vi "Render Section.vi"(6 "Loader":refnum<class "Loader.lvclass">, 8 "Error In":errorcluster, 10 "Section":refnum<class "Section.lvclass">, 11 "Context In":refnum<class "Context.lvclass">) -> (0 "Error Out":errorcluster, 2 "Output":string, 3 "Context Out":refnum<class "Context.lvclass">)   [LabVIEW 2018, in "Toolkit.lvlib"]
uses:
  Toolkit.lvlib
  Context/Context.lvclass
  Nodes/Section/Section.lvclass
  Loaders/Loader/Loader.lvclass
  Nodes/Section/Section.lvclass/Section.ctl
  Data/Array/Array.lvclass
  Data/Array/Array.lvclass/Array.ctl
  Context/Context.lvclass/Context.ctl
  Data/Boolean/Boolean.lvclass
  Data/Function/Function.lvclass
  Data/String/String.lvclass
  Data/String/String.lvclass/String.ctl
  Data/Path/Path.lvclass
  Data/Path/Path.lvclass/Path.ctl
  Data/Datum/Datum.lvclass
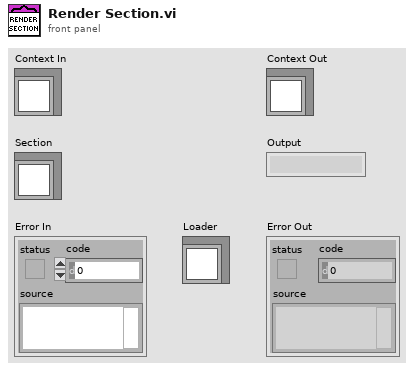
[diagram p1: front panel]
types:
  T1 = typedef "Toolkit.lvlib/Data.lvlib/Types.ctl" = enum16{"Array", "Boolean", "Function", "Map", "Null", "Pair", "Path", "String", "Unknown"}
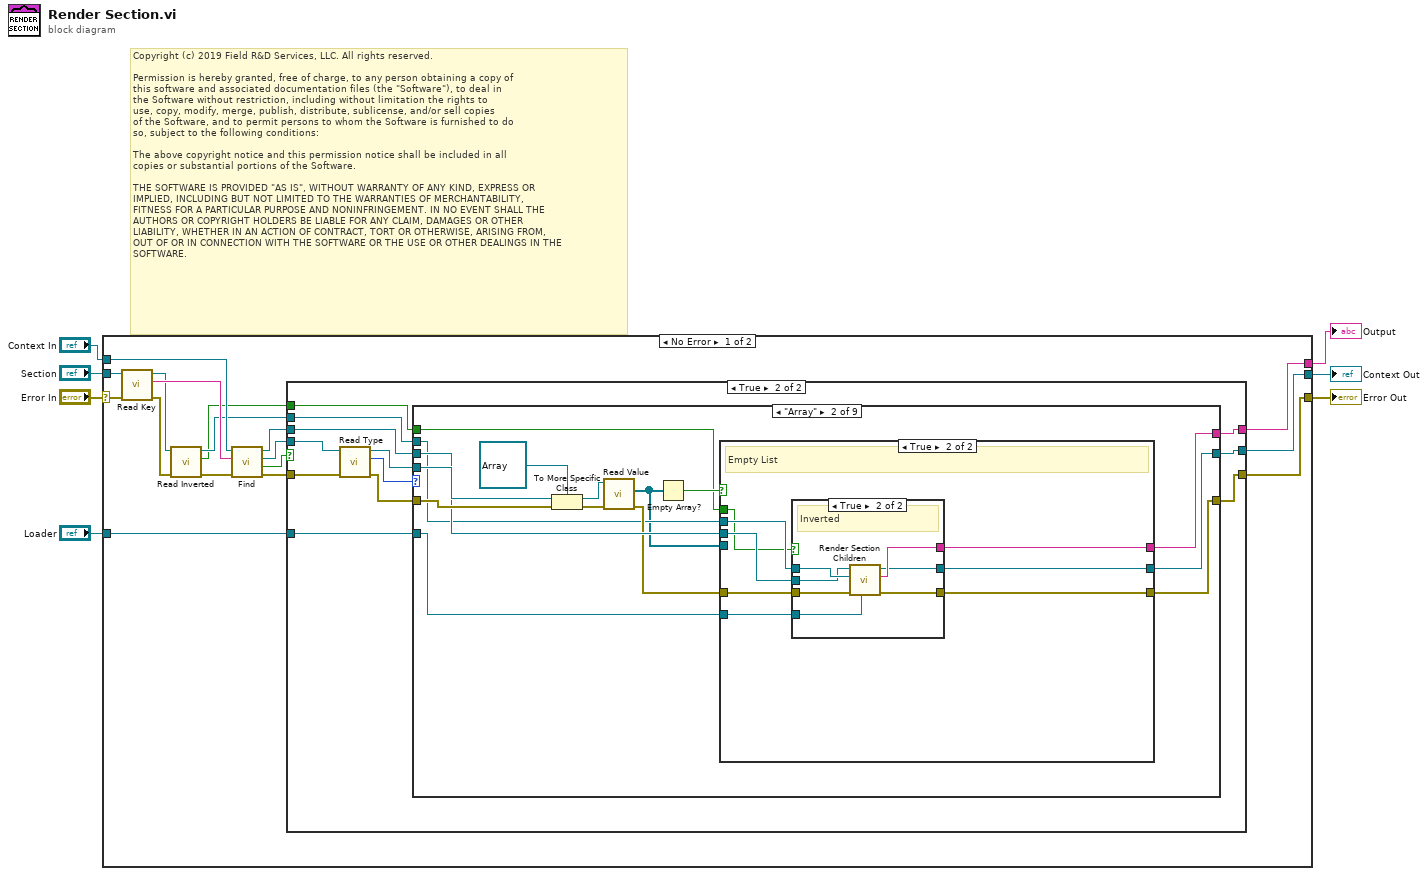
[diagram p0: block diagram]
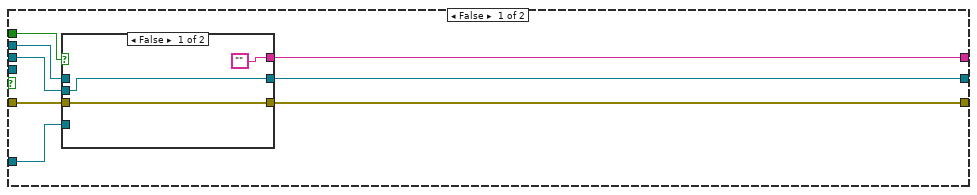
[diagram p2: hidden frame]
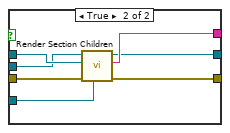
[diagram p3: hidden frame]
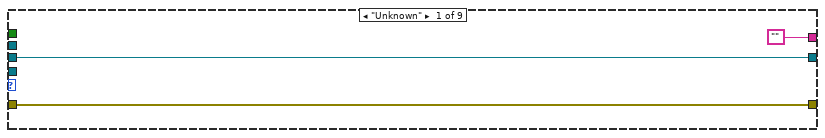
[diagram p4: hidden frame]
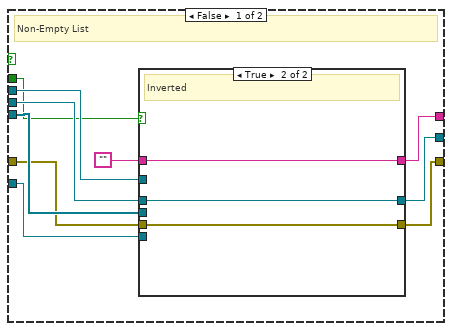
[diagram p5: hidden frame]
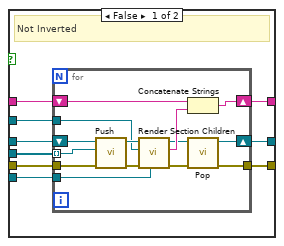
[diagram p6: hidden frame]
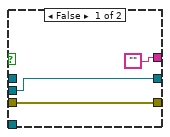
[diagram p7: hidden frame]
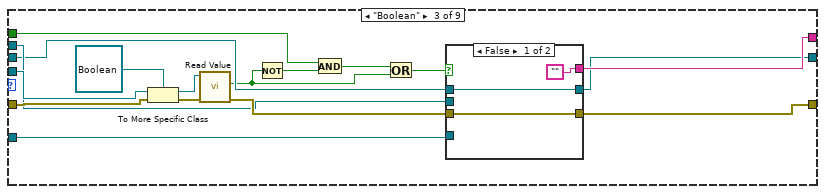
[diagram p8: hidden frame]
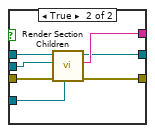
[diagram p9: hidden frame]
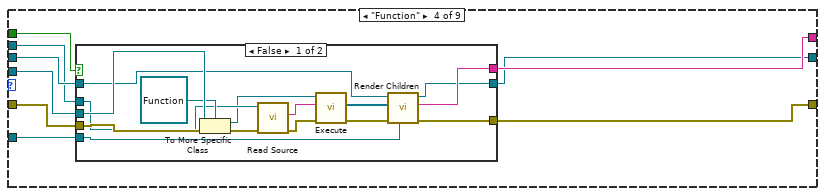
[diagram p10: hidden frame]
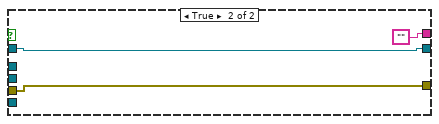
[diagram p11: hidden frame]
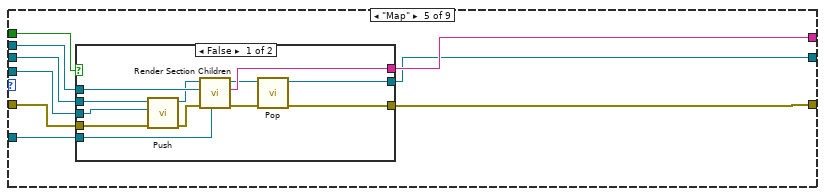
[diagram p12: hidden frame]
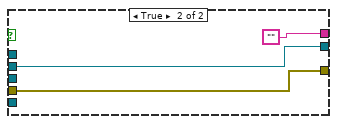
[diagram p13: hidden frame]
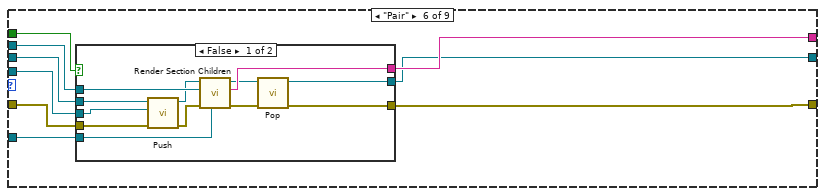
[diagram p14: hidden frame]
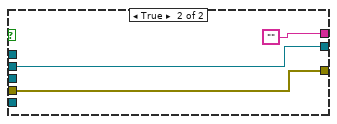
[diagram p15: hidden frame]
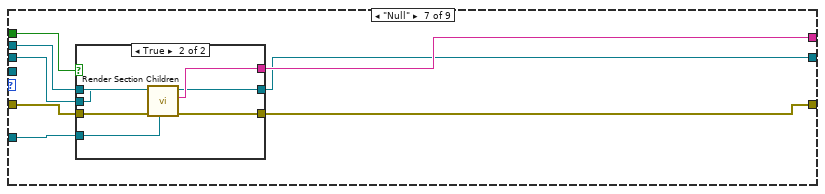
[diagram p16: hidden frame]
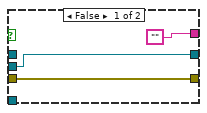
[diagram p17: hidden frame]
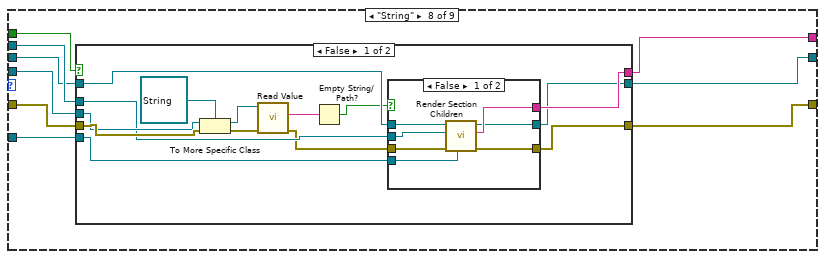
[diagram p18: hidden frame]
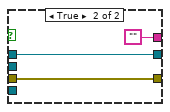
[diagram p19: hidden frame]
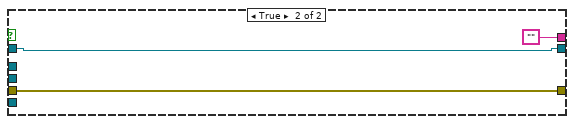
[diagram p20: hidden frame]
diagram:
  # "Copyright (c) 2019 Field R&D Services, LLC. All rights reserved.\n\nPermission is hereby granted, free of charge, to any person obtaining a copy of\nthis software and associated documentation files (the \"Software\"), to deal in\nthe Software without restriction, including without limitation the rights to\nuse, copy, modify, merge, publish, distribute, sublicense, and/or sell copies\nof the Software, and to permit persons to whom the Software is furnished to do\nso, subject to the following conditions:\n\nThe above copyright notice and this permission notice shall be included in all\ncopies or substantial portions of the Software.\n\nTHE SOFTWARE IS PROVIDED \"AS IS\", WITHOUT WARRANTY OF ANY KIND, EXPRESS OR\nIMPLIED, INCLUDING BUT NOT LIMITED TO THE WARRANTIES OF MERCHANTABILITY,\nFITNESS FOR A PARTICULAR PURPOSE AND NONINFRINGEMENT. IN NO EVENT SHALL THE\nAUTHORS OR COPYRIGHT HOLDERS BE LIABLE FOR ANY CLAIM, DAMAGES OR OTHER\nLIABILITY, WHETHER IN AN ACTION OF CONTRACT, TORT OR OTHERWISE, ARISING FROM,\nOUT OF OR IN CONNECTION WITH THE SOFTWARE OR THE USE OR OTHER DEALINGS IN THE\nSOFTWARE."
  n1 = case shown="No Error" "Error In" {
    selector: "Error In" -> [w17 w323]
    tunnel: "Section" -> [w16 _]
    tunnel: [w21 w323] -> w6
    tunnel: [w22 ""] -> w5
    tunnel: "Context In" -> [w24 w321]
    tunnel: [w9 w321] -> w2
    tunnel: "Loader" -> [w8 _]
    frame No Error {
      n2 = call "Read Key.vi"("Error In"=w17, "Section In"=w16) -> ("Error Out"=w12:errorcluster, "Key"=w15:string, "Section Out"=w14:refnum<class "Section.lvclass">)  [unwired: 7 in]
      n3 = call "Read Inverted.vi"("Error In"=w12, "Section In"=w14) -> ("Error Out"=w11:errorcluster, "Inverted"=w10:bool, "Section Out"=w13:refnum<class "Section.lvclass">)  [unwired: 7 in]
      n4 = call "Find.vi"("Error In"=w11, "Key"=w15, "Context In"=w24) -> ("Error Out"=w20:errorcluster, "Found?"=w23:bool, "Datum"=w19:refnum<class "Datum.lvclass">, "Context Out"=w18:refnum<class "Context.lvclass">)  [unwired: 5 in]
      n5 = case shown="True" w23 {
        tunnel: [w27 w54] -> w22
        tunnel: [w31 w53] -> w21
        tunnel: w20 -> [w32 w45]
        tunnel: w19 -> [_ w52]
        tunnel: w13 -> [w30 w51]
        tunnel: w18 -> [w28 w50]
        tunnel: w10 -> [w29 w49]
        tunnel: [w26 w48] -> w9
        tunnel: w8 -> [w25 w43]
        frame False {
          n6 = case shown="False" w29 {
            tunnel: w32 -> [w34 w42]
            tunnel: [w34 w41] -> w31
            tunnel: w30 -> [_ w40]
            tunnel: ["" w39] -> w27
            tunnel: w28 -> [w33 w38]
            tunnel: [w33 w37] -> w26
            tunnel: w25 -> [_ w36]
            frame False {
            }
            frame True {
              n7 = call "Render Section Children.vi"("Loader"=w36, "Error In"=w42, "Section"=w40, "Context In"=w38) -> ("Error Out"=w41:errorcluster, "Output"=w39:string, "Context Out"=w37:refnum<class "Context.lvclass">)  [unwired: 5 in]
            }
          }
        }
        frame True {
          n8 = call-dynamic "Read Type.vi"("Error In"=w45, "Datum In"=w52) -> ("Error Out"=w44:errorcluster, "Type"=w46:T1, "Datum Out"=w47:refnum<class "Datum.lvclass">)  [unwired: 7 in]
          n9 = case shown="\"Array\"" w46 {
            tunnel: w44 -> [w57 w72 w143 w162 w185 w209 w235 w255 w291]
            tunnel: ["" w64 w138 w158 w184 w208 w232 w253 w289] -> w54
            tunnel: [w57 w65 w137 w159 w188 w212 w234 w252 w288] -> w53
            tunnel: w47 -> [_ w71 w142 w161 w186 w210 _ w254 w290]
            tunnel: w51 -> [_ w63 w136 w157 w187 w211 w233 w251 w287]
            tunnel: w50 -> [w55 w67 w135 w160 w189 w213 w231 w250 w286]
            tunnel: w49 -> [_ w58 w131 w156 w183 w207 w236 w249 w285]
            tunnel: [w55 w61 w129 w155 w182 w206 w230 w248 w284] -> w48
            tunnel: w43 -> [_ w60 w127 w154 w181 w205 w229 w247 w283]
            frame "Unknown" {
            }
            frame "Array" {
              n10 = To More Specific Class(target class=refnum<class "Array.lvclass"> refnum ("Toolkit.lvlib:Data.lvlib:Array.lvclass"), reference=w71, error in=w72) -> (specific class reference=w69:refnum<class "Array.lvclass">, error out=w68:errorcluster)
              n11 = call "Read Value.vi"("Error In"=w68, "Array In"=w69) -> ("Error Out"=w66:errorcluster, "Value"=w62:refnum<class "Datum.lvclass">[])  [unwired: 7 in, 1 out]
              n12 = Empty Array?(array=w62) -> (empty?=w59:bool)
              n13 = case shown="True" w59 {
                tunnel: w62 -> [w82 _]
                tunnel: w67 -> [w81 w112]
                tunnel: w66 -> [w80 w114]
                tunnel: [w79 w113] -> w65
                tunnel: [w78 w115] -> w64
                tunnel: w63 -> [w76 w116]
                tunnel: [w77 w111] -> w61
                tunnel: w60 -> [w75 w110]
                tunnel: w58 -> [w74 w109]
                frame False {
                  # "Non-Empty List"
                  n14 = case shown="True" w74 {
                    tunnel: w82 -> [w91 _]
                    tunnel: w81 -> [w90 w107]
                    tunnel: w80 -> [w89 w106]
                    tunnel: [w88 w106] -> w79
                    tunnel: [w87 w108] -> w78
                    tunnel: [w86 w107] -> w77
                    tunnel: w76 -> [w85 _]
                    tunnel: w75 -> [w84 _]
                    tunnel: "" -> [w83 w108]
                    frame False {
                      # "Not Inverted"
                      n15 = for {
                        tunnel: w91 -> [w103] mode=indexing
                        tunnel: w89 -> [w105]
                        shift-right: [w102] -> w86
                        shift-left: w90 -> [w104]
                        tunnel: [w101] -> w88
                        shift-right: [w99] -> w87
                        shift-left: w83 -> [w100]
                        tunnel: w85 -> [w93]
                        tunnel: w84 -> [w92]
                        n16 = call "Push.vi"("Error In"=w105, "Datum"=w103, "Context In"=w104) -> ("Error Out"=w97:errorcluster, "Context Out"=w98:refnum<class "Context.lvclass">)  [unwired: 7 in]
                        n17 = call "Render Section Children.vi"("Loader"=w92, "Error In"=w97, "Section"=w93, "Context In"=w98) -> ("Error Out"=w96:errorcluster, "Output"=w95:string, "Context Out"=w94:refnum<class "Context.lvclass">)  [unwired: 5 in]
                        n18 = Concatenate Strings(w100, w95) -> (w99:string)
                        n19 = call "Pop.vi"("Error In"=w96, "Context In"=w94) -> ("Error Out"=w101:errorcluster, "Context Out"=w102:refnum<class "Context.lvclass">)  [unwired: 7 in, 1 out]
                      }
                    }
                    frame True {
                      # "Inverted"
                    }
                  }
                }
                frame True {
                  # "Empty List"
                  n20 = case shown="True" w109 {
                    tunnel: w116 -> [_ w126]
                    tunnel: ["" w125] -> w115
                    tunnel: w114 -> [w118 w124]
                    tunnel: [w118 w123] -> w113
                    tunnel: w112 -> [w119 w122]
                    tunnel: [w119 w121] -> w111
                    tunnel: w110 -> [_ w120]
                    frame False {
                    }
                    frame True {
                      # "Inverted"
                      n21 = call "Render Section Children.vi"("Loader"=w120, "Error In"=w124, "Section"=w126, "Context In"=w122) -> ("Error Out"=w123:errorcluster, "Output"=w125:string, "Context Out"=w121:refnum<class "Context.lvclass">)  [unwired: 5 in]
                    }
                  }
                }
              }
            }
            frame "Boolean" {
              n22 = To More Specific Class(target class=refnum<class "Boolean.lvclass"> refnum ("Toolkit.lvlib:Data.lvlib:Boolean.lvclass"), reference=w142, error in=w143) -> (specific class reference=w128:refnum<class "Boolean.lvclass">, error out=w140:errorcluster)
              n23 = call "Read Value.vi"("Error In"=w140, "Boolean In"=w128) -> ("Error Out"=w139:errorcluster, "Value"=w134:bool)  [unwired: 7 in, 1 out]
              n24 = Not(x=w134) -> (.not. x?=w133:bool)
              n25 = And(x=w131, y=w133) -> (x .and. y?=w132:bool)
              n26 = Or(x=w132, y=w134) -> (x .or. y?=w130:bool)
              n27 = case shown="False" w130 {
                tunnel: w139 -> [w145 w153]
                tunnel: ["" w150] -> w138
                tunnel: [w145 w151] -> w137
                tunnel: w136 -> [_ w152]
                tunnel: w135 -> [w144 w149]
                tunnel: [w144 w148] -> w129
                tunnel: w127 -> [_ w147]
                frame False {
                }
                frame True {
                  n28 = call "Render Section Children.vi"("Loader"=w147, "Error In"=w153, "Section"=w152, "Context In"=w149) -> ("Error Out"=w151:errorcluster, "Output"=w150:string, "Context Out"=w148:refnum<class "Context.lvclass">)  [unwired: 5 in]
                }
              }
            }
            frame "Function" {
              n29 = case shown="False" w156 {
                tunnel: w162 -> [w177 w180]
                tunnel: w161 -> [w176 _]
                tunnel: w160 -> [w166 w178]
                tunnel: [w173 w180] -> w159
                tunnel: [w172 ""] -> w158
                tunnel: w157 -> [w171 _]
                tunnel: [w165 w178] -> w155
                tunnel: w154 -> [w163 _]
                frame False {
                  n30 = To More Specific Class(target class=refnum<class "Function.lvclass"> refnum ("Toolkit.lvlib:Data.lvlib:Function.lvclass"), reference=w176, error in=w177) -> (specific class reference=w164:refnum<class "Function.lvclass">, error out=w169:errorcluster)
                  n31 = call-dynamic "Read Source.vi"("Error In"=w169, "Node In"=w171) -> ("Error Out"=w168:errorcluster, "Source"=w167:string)  [unwired: 7 in, 1 out]
                  n32 = call-dynamic "Execute.vi"("Error In"=w168, "Source"=w167, "Function In"=w164) -> ("Error Out"=w170:errorcluster, "Nodes"=w174:refnum<class "Node.lvclass">[])  [unwired: 6 in, 1 out]
                  n33 = call "Render Children.vi"("Loader"=w163, "Error In"=w170, "Children"=w174, "Context In"=w166) -> ("Error Out"=w173:errorcluster, "Output"=w172:string, "Context Out"=w165:refnum<class "Context.lvclass">)  [unwired: 5 in]
                }
                frame True {
                }
              }
            }
            frame "Map" {
              n34 = case shown="False" w183 {
                tunnel: w189 -> [w201 w202]
                tunnel: [w200 w204] -> w188
                tunnel: w187 -> [w199 _]
                tunnel: w186 -> [w195 _]
                tunnel: w185 -> [w194 w204]
                tunnel: [w193 ""] -> w184
                tunnel: [w192 w202] -> w182
                tunnel: w181 -> [w190 _]
                frame False {
                  n35 = call "Push.vi"("Error In"=w194, "Datum"=w195, "Context In"=w201) -> ("Error Out"=w197:errorcluster, "Context Out"=w198:refnum<class "Context.lvclass">)  [unwired: 7 in]
                  n36 = call "Render Section Children.vi"("Loader"=w190, "Error In"=w197, "Section"=w199, "Context In"=w198) -> ("Error Out"=w196:errorcluster, "Output"=w193:string, "Context Out"=w191:refnum<class "Context.lvclass">)  [unwired: 5 in]
                  n37 = call "Pop.vi"("Error In"=w196, "Context In"=w191) -> ("Error Out"=w200:errorcluster, "Context Out"=w192:refnum<class "Context.lvclass">)  [unwired: 7 in, 1 out]
                }
                frame True {
                }
              }
            }
            frame "Pair" {
              n38 = case shown="False" w207 {
                tunnel: w213 -> [w225 w226]
                tunnel: [w224 w228] -> w212
                tunnel: w211 -> [w223 _]
                tunnel: w210 -> [w219 _]
                tunnel: w209 -> [w218 w228]
                tunnel: [w217 ""] -> w208
                tunnel: [w216 w226] -> w206
                tunnel: w205 -> [w214 _]
                frame False {
                  n39 = call "Push.vi"("Error In"=w218, "Datum"=w219, "Context In"=w225) -> ("Error Out"=w221:errorcluster, "Context Out"=w222:refnum<class "Context.lvclass">)  [unwired: 7 in]
                  n40 = call "Render Section Children.vi"("Loader"=w214, "Error In"=w221, "Section"=w223, "Context In"=w222) -> ("Error Out"=w220:errorcluster, "Output"=w217:string, "Context Out"=w215:refnum<class "Context.lvclass">)  [unwired: 5 in]
                  n41 = call "Pop.vi"("Error In"=w220, "Context In"=w215) -> ("Error Out"=w224:errorcluster, "Context Out"=w216:refnum<class "Context.lvclass">)  [unwired: 7 in, 1 out]
                }
                frame True {
                }
              }
            }
            frame "Null" {
              n42 = case shown="True" w236 {
                tunnel: w235 -> [w238 w246]
                tunnel: [w238 w245] -> w234
                tunnel: w233 -> [_ w244]
                tunnel: ["" w243] -> w232
                tunnel: w231 -> [w237 w242]
                tunnel: [w237 w241] -> w230
                tunnel: w229 -> [_ w240]
                frame False {
                }
                frame True {
                  n43 = call "Render Section Children.vi"("Loader"=w240, "Error In"=w246, "Section"=w244, "Context In"=w242) -> ("Error Out"=w245:errorcluster, "Output"=w243:string, "Context Out"=w241:refnum<class "Context.lvclass">)  [unwired: 5 in]
                }
              }
            }
            frame "String" {
              n44 = case shown="False" w249 {
                tunnel: w255 -> [w269 w282]
                tunnel: w254 -> [w268 _]
                tunnel: [w267 ""] -> w253
                tunnel: [w266 w282] -> w252
                tunnel: w251 -> [w265 _]
                tunnel: w250 -> [w264 w280]
                tunnel: [w257 w280] -> w248
                tunnel: w247 -> [w256 _]
                frame False {
                  n45 = To More Specific Class(target class=refnum<class "String.lvclass"> refnum ("Toolkit.lvlib:Data.lvlib:String.lvclass"), reference=w268, error in=w269) -> (specific class reference=w261:refnum<class "String.lvclass">, error out=w262:errorcluster)
                  n46 = call "Read Value.vi"("Error In"=w262, "String In"=w261) -> ("Error Out"=w258:errorcluster, "Value"=w260:string)  [unwired: 7 in, 1 out]
                  n47 = Empty String/Path?(string/path=w260) -> (empty?=w259:bool)
                  n48 = case shown="False" w259 {
                    tunnel: [w274 ""] -> w267
                    tunnel: [w275 w278] -> w266
                    tunnel: w265 -> [w276 _]
                    tunnel: w264 -> [w272 w277]
                    tunnel: w258 -> [w273 w278]
                    tunnel: [w271 w277] -> w257
                    tunnel: w256 -> [w270 _]
                    frame False {
                      n49 = call "Render Section Children.vi"("Loader"=w270, "Error In"=w273, "Section"=w276, "Context In"=w272) -> ("Error Out"=w275:errorcluster, "Output"=w274:string, "Context Out"=w271:refnum<class "Context.lvclass">)  [unwired: 5 in]
                    }
                    frame True {
                    }
                  }
                }
                frame True {
                }
              }
            }
            frame "Path" {
              n50 = case shown="False" w285 {
                tunnel: w291 -> [w307 w320]
                tunnel: w290 -> [w306 _]
                tunnel: [w305 ""] -> w289
                tunnel: [w304 w320] -> w288
                tunnel: w287 -> [w303 _]
                tunnel: w286 -> [w302 w318]
                tunnel: [w298 w318] -> w284
                tunnel: w283 -> [w292 _]
                frame False {
                  n51 = To More Specific Class(target class=refnum<class "Path.lvclass"> refnum ("Toolkit.lvlib:Data.lvlib:Path.lvclass"), reference=w306, error in=w307) -> (specific class reference=w300:refnum<class "Path.lvclass">, error out=w301:errorcluster)
                  n52 = call "Read Value.vi"("Error In"=w301, "Path In"=w300) -> ("Error Out"=w299:errorcluster, "Value"=w294:path)  [unwired: 7 in, 1 out]
                  n53 = Not A Number/Path/Refnum?(number/path/refnum=w294) -> (NaN/Path/Refnum?=w295:bool)
                  n54 = Empty String/Path?(string/path=w294) -> (empty?=w296:bool)
                  n55 = Compound Arithmetic op=OR(w295, w296) -> (invert w293:bool)
                  n56 = case shown="True" w293 {
                    tunnel: ["" w315] -> w305
                    tunnel: [w309 w316] -> w304
                    tunnel: w303 -> [_ w317]
                    tunnel: w302 -> [w308 w313]
                    tunnel: w299 -> [w309 w314]
                    tunnel: [w308 w312] -> w298
                    tunnel: w292 -> [_ w311]
                    frame False {
                    }
                    frame True {
                      n57 = call "Render Section Children.vi"("Loader"=w311, "Error In"=w314, "Section"=w317, "Context In"=w313) -> ("Error Out"=w316:errorcluster, "Output"=w315:string, "Context Out"=w312:refnum<class "Context.lvclass">)  [unwired: 5 in]
                    }
                  }
                }
                frame True {
                }
              }
            }
          }
        }
      }
    }
    frame Error {
    }
  }
  "Error Out" <- w6
  "Output" <- w5
  "Context Out" <- w2
